vi "090812_MotorC84320_Test.vi"() -> ()   [LabVIEW 2010]
panel:
  out "+/- movement\nrange":dbl[](array[numeric]) format="%.6f"
  out "Position":dbl[](array[numeric]) format="%.6f"
  out "Boolean":bool
  in  "stop":bool
  out "Axis on target?":bool[](array[boolean])
  in  "Position values":dbl[](array[numeric]) format="%.6f"
  in  "Use dialog to define\nconnected stages?":bool=TRUE
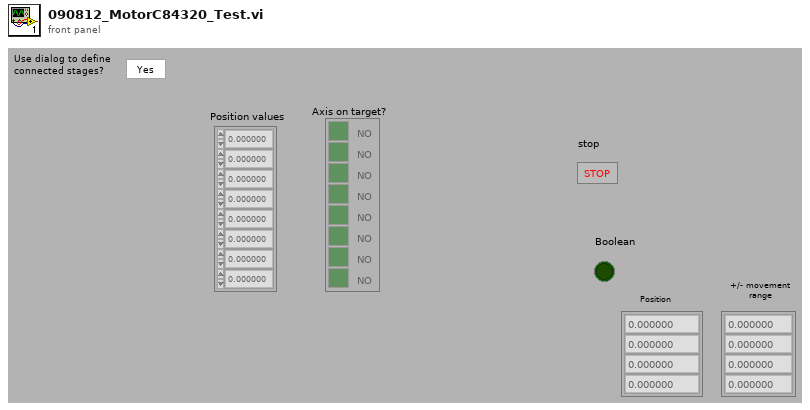
[diagram p1: front panel]
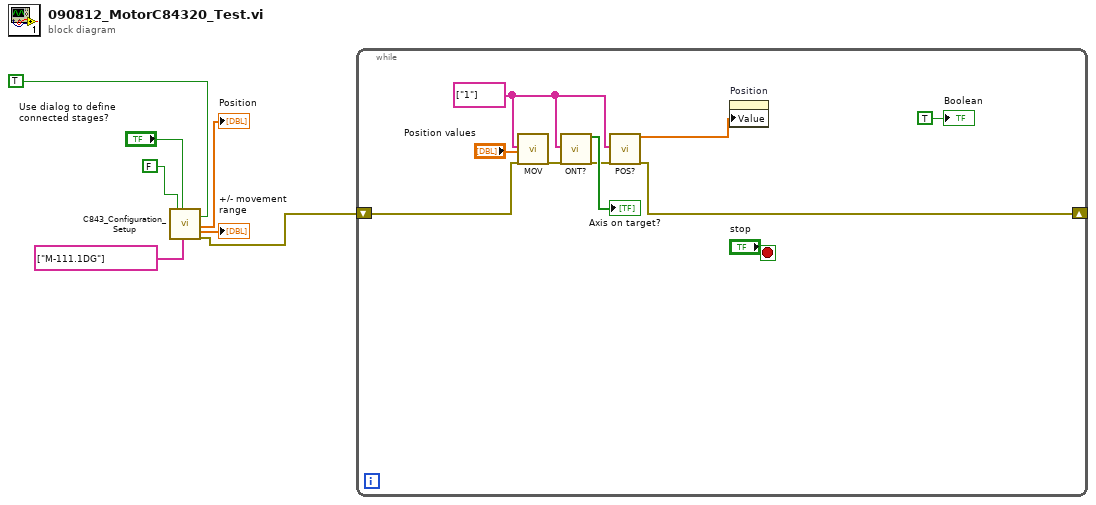
[diagram p0: block diagram]
diagram:
  n1 = call "C843_Configuration_Setup.vi"("C-843 version"=FALSE, "Use dialog to define\nconnected stages?"="Use dialog to define\nconnected stages?", "Stage names input"=string[] ["M-111.1DG"], "Move to middle?"=TRUE) -> ("Position"=→"Position":dbl[], "+/- movement\nrange"=→"+/- movement\nrange":dbl[], "error out"=w5:errorcluster)  [unwired: 11 in, 2 out]
  n2 = while {
    shift-right: [w10] -> _
    shift-left: w5 -> [w17]
    stop <- "stop" stop-if-true
    w9 = string[] ["1"] ("Axes to move")
    n3 = call "MOV.vi"("Axes to move"=w9, "Position values"="Position values", "error in"=w17) -> ("error out"=w15:errorcluster)  [unwired: 16 in]
    n4 = call "ONT?.vi"("Axes to query"=w9, "error in"=w15) -> ("Axis on target?"=→"Axis on target?":bool[], "error out"=w11:errorcluster)  [unwired: 16 in]
    n5 = call "POS?.vi"("Axes to query"=w9, "error in"=w11) -> ("Position"=w8:dbl[], "error out"=w10:errorcluster)  [unwired: 16 in]
    n6 = property on="Position" class="Arr (strict)"("Value"=w8) -> ()  [unwired: 2 in, 2 out]
    "Boolean" <- TRUE ("Boolean")
  }
